vi "Update_library.vi"(1 "Librairie des objets":string[][](table)=[["1", "WR1", "00:43:28", "64:45:35", "2000.0", "1.153488"], ["2", "WR2", "01:05:23", "60:25:18", "2000.0", "1.142985"], ["3", "WR3", "02:54:30", "-10:00:17", "2006.2", "2.742240"], ["4", "WR4", "02:00:00", "10:00:00", "2000.0", "1.613543"], ["5", "WR5", "02:52:11", "56:56:07", "2000.0", "1.148727"], ["6", "WR6", "06:54:13", "-23:55:42", "2000.0", "7.346970"], ["7", "WR7", "07:18:29", "-13:13:01", "2000.0", "3.540250"], ["8", "WR7a", "07:20:22", "-23:43:57", "2000.0", "7.387993"], ["9", "WR8", "07:44:58", "-31:54:29", "2000.0", "29.253050"]], 2 "String to Search":string) -> (0 "lib_out":string[][](table)=[["1", "WR1", "00:43:28", "64:45:35", "2000.0", "1.153488"], ["2", "WR2", "01:05:23", "60:25:18", "2000.0", "1.142985"], ["3", "WR3", "02:54:30", "-10:00:17", "2006.2", "2.742240"], ["4", "WR4", "02:00:00", "10:00:00", "2000.0", "1.613543"], ["5", "WR5", "02:52:11", "56:56:07", "2000.0", "1.148727"], ["6", "WR6", "06:54:13", "-23:55:42", "2000.0", "7.346970"], ["7", "WR7", "07:18:29", "-13:13:01", "2000.0", "3.540250"], ["8", "WR7a", "07:20:22", "-23:43:57", "2000.0", "7.387993"], ["9", "WR8", "07:44:58", "-31:54:29", "2000.0", "29.253050"]])   [LabVIEW 2019]
panel:
  out "Array":bool[](array[boolean])
  out "rm":i32[](array[numeric])
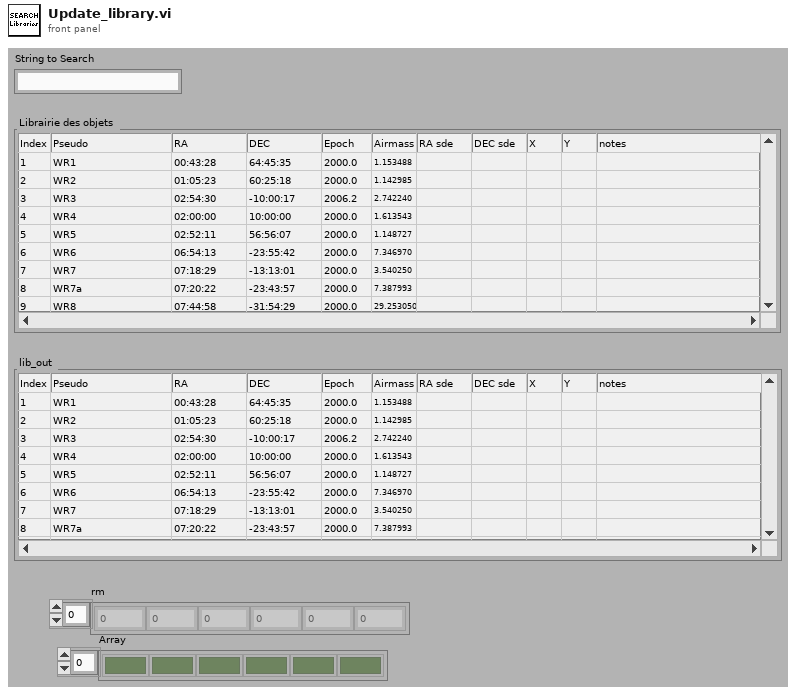
[diagram p1: front panel]
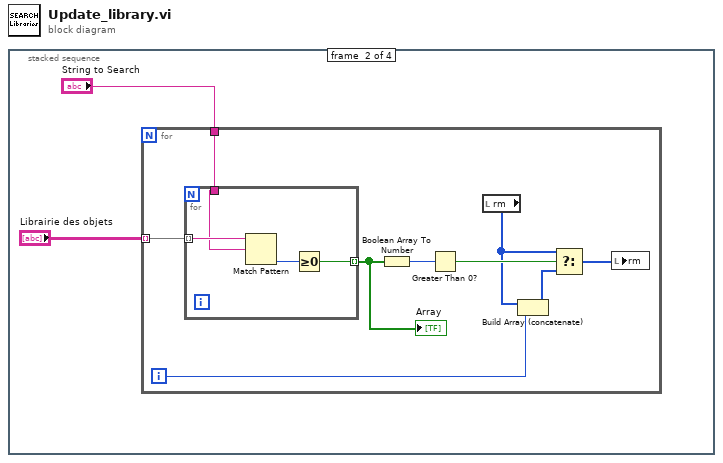
[diagram p0: block diagram]
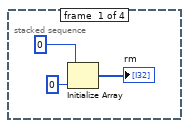
[diagram p2: hidden frame]
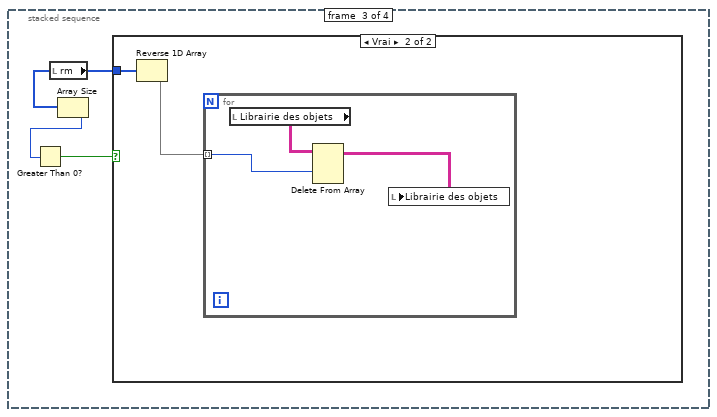
[diagram p3: hidden frame]
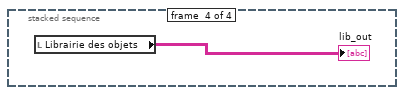
[diagram p5: hidden frame]
diagram:
  n1 = stacked-sequence {
    frame #0 {
      n2 = Initialize Array(0, 0 ("dimension size")) -> (→"rm":i32[])
    }
    frame #1 {
      n3 = for {
        tunnel: "Librairie des objets" -> [w7] mode=indexing
        tunnel: "String to Search" -> [w14]
        i -> [w9]
        n4 = for {
          tunnel: w14 -> [w15]
          tunnel: [w17] -> w6 mode=indexing
          tunnel: w7 -> [w16] mode=indexing
          n5 = Match Pattern(string=w16, regular expression=w15) -> (offset past match=w18:i32)  [unwired: 1 in, 3 out]
          n6 = Greater Or Equal To 0?(x=w18) -> (x >= 0?=w17:bool)
        }
        "Array" <- w6
        n7 = Boolean Array To Number(Boolean array=w6) -> (number=w13:u32)
        n8 = Greater Than 0?(x=w13) -> (x > 0?=w12:bool)
        n9 = local read "rm"() -> (w10:i32[])
        n10 = Build Array (concatenate)(w10, w9) -> (w8:i32[])
        n11 = Select(t=w10, s=w12, f=w8) -> (s? t:f=w11:i32[])
        n12 = local write "rm"(w11) -> ()
      }
    }
    frame #2 {
      n13 = local read "rm"() -> (w19:i32[])
      n14 = Array Size(array=w19) -> (size(s)=w21:i32)
      n15 = Greater Than 0?(x=w21) -> (x > 0?=w20:bool)
      n16 = case shown="Vrai" w20 {
        tunnel: w19 -> [_ w23]
        frame False {
        }
        frame True {
          n17 = Reverse 1D Array(array=w23) -> (reversed array=w22:i32[])
          n18 = for {
            tunnel: w22 -> [w25] mode=indexing
            n19 = local read "Librairie des objets"() -> (w26:string[][])
            n20 = Delete From Array(array=w26, index (row)=w25) -> (array with subset deleted=w24:string[][])  [unwired: 2 in, 1 out]
            n21 = local write "Librairie des objets"(w24) -> ()
          }
        }
      }
    }
    frame #3 {
      n22 = local read "Librairie des objets"() -> (→"lib_out":string[][])
    }
  }
